vi "FTIR_multiple.vi"() -> ()   [LabVIEW 2021]
uses:
  <vilib>/express/express analysis/Spectral/Block/exnSpectralBlock spectral measurements PSD poly.vi
  <vilib>/express/express analysis/Spectral/Block/exnSpectralBlock spectral measurements PSD DDT.vi
  <vilib>/express/express analysis/Spectral/XNode/ExpressSpectralMeasurementsBlockNode.xnode
panel:
  out "Interferogram frequency":dbl[](array[numeric])
  out "Interferogram":dynamicdata(graph)
  out "FFT interferogram":dynamicdata(graph)
  out "Waveform signal":dynamicdata(graph)
  in  "Mirror 1 distance":dbl
  out "Phase":dbl[](array[numeric])
  out "size(s)":i32
  in  "Mirror speed":dbl(slide) scale=0.0..0.3
  out "Frequency 2":dbl[](array[numeric])
  out "Frequency 1":dbl[](array[numeric])
  out "Wavenumber":dbl[](array[numeric])
  in  "Wavelength":dbl[](array[numeric])
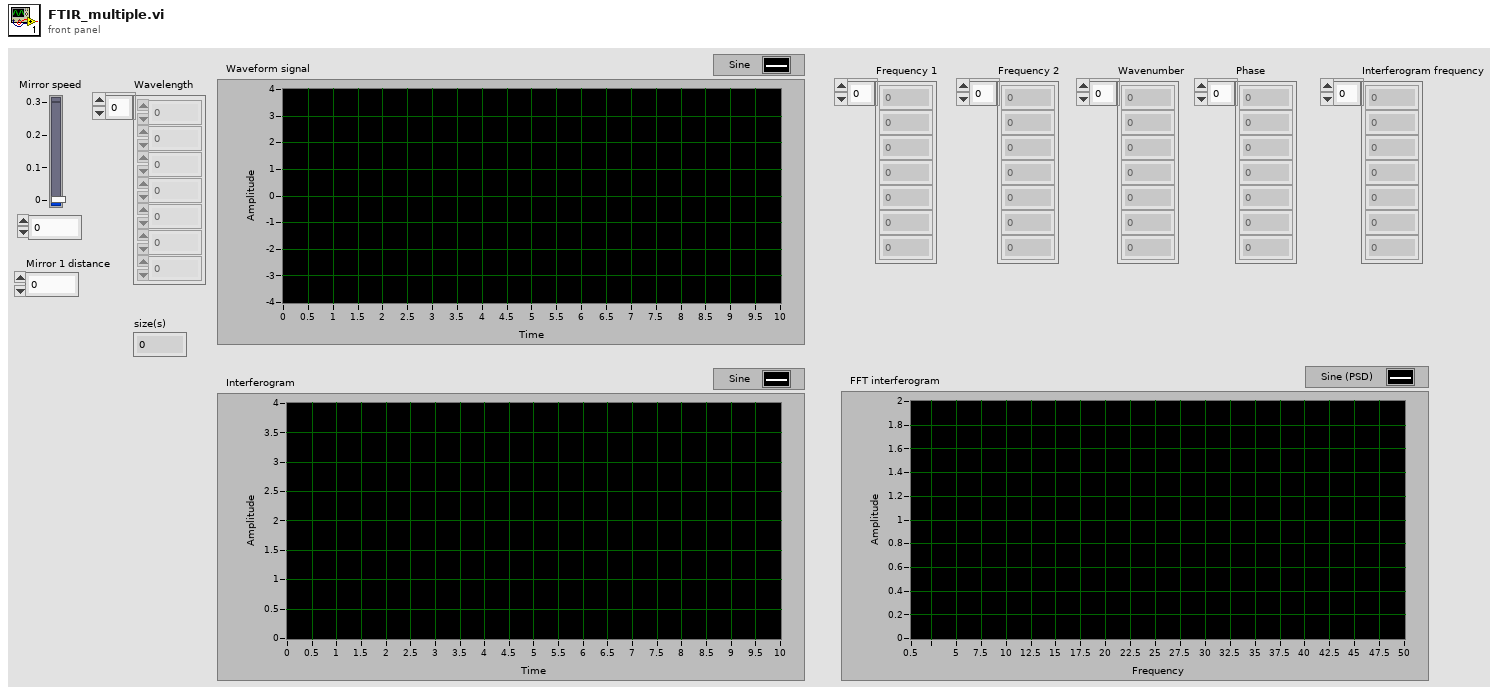
[diagram p1: front panel]
types:
  T1 = cluster{"averaging mode":u16, "weighting mode":u16, "number of averages":u32}
  T2 = cluster{"dB On (F)":bool, "unwrap phase (F)":bool, "convert to degree (F)":bool}
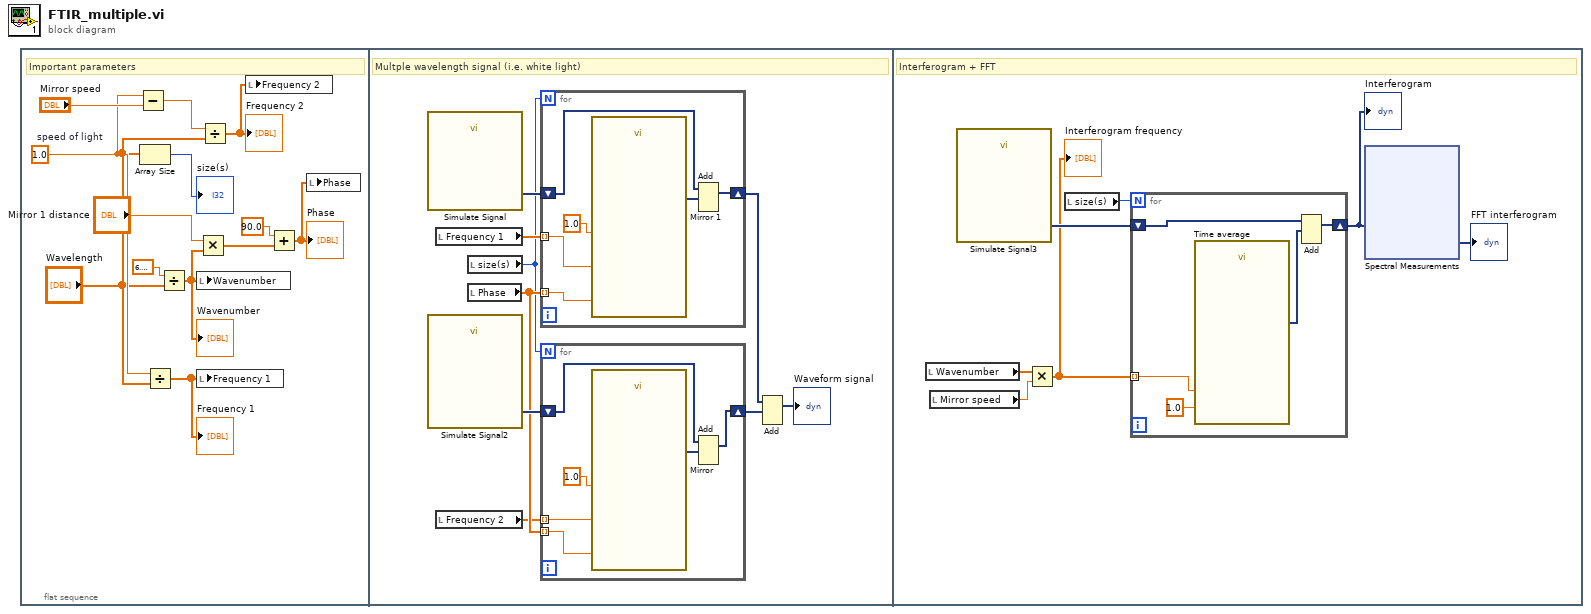
[diagram p0: block diagram]
diagram:
  n1 = flat-sequence {
    frame #0 {
      w11 = 1.0  # speed of light
      # "Important parameters"
      n2 = Subtract(x=w11, y="Mirror speed") -> (x-y=w13:dbl)
      n3 = Array Size(array="Wavelength") -> (size(s)=→"size(s)":i32)
      n4 = Divide(x=w11, y="Wavelength") -> (x/y=w6:dbl[])
      "Frequency 1" <- w6
      n5 = Divide(x=6.283185307179586, y="Wavelength") -> (x/y=w7:dbl[])
      "Wavenumber" <- w7
      n6 = local write "Wavenumber"(w7) -> ()
      n7 = local write "Frequency 1"(w6) -> ()
      n8 = Multiply(x="Mirror 1 distance", y=w7) -> (x*y=w9:dbl[])
      n9 = Divide(x=w13, y="Wavelength") -> (x/y=w5:dbl[])
      "Frequency 2" <- w5
      n10 = local write "Frequency 2"(w5) -> ()
      n11 = Add(x=90.0 ("y"), y=w9) -> (x+y=w2:dbl[])
      "Phase" <- w2
      n12 = local write "Phase"(w2) -> ()
    }
    frame #1 {
      # "Multple wavelength signal (i.e. white light)"
      n13 = call "Simulate Signal"() -> ("Sine"=w21:dynamicdata)  [unwired: 14 in, 1 out]
      n14 = call "Simulate Signal2"() -> ("Sine"=w20:dynamicdata)  [unwired: 14 in, 1 out]
      n15 = local read "Frequency 1"() -> (w22:dbl[])
      n16 = local read "Frequency 2"() -> (w17:dbl[])
      n17 = local read "size(s)"() -> (w18:i32)
      n18 = local read "Phase"() -> (w19:dbl[])
      n19 = for {
        N: w18 -> [_]
        tunnel: w22 -> [w34] mode=indexing
        tunnel: w19 -> [w33] mode=indexing
        shift-right: [w30] -> w16
        shift-left: w21 -> [w31]
        n20 = call "Mirror 1"("Frequency"=w34, "Amplitude"=1.0, "Phase"=w33) -> ("Sine"=w32:dynamicdata)  [unwired: 11 in, 1 out]
        n21 = Add(1:w32, 2:w31) -> (0:w30:dynamicdata)  [unwired: 1 in, 1 out]
      }
      n22 = for {
        N: w18 -> [_]
        shift-right: [w26] -> w15
        shift-left: w20 -> [w27]
        tunnel: w19 -> [w25] mode=indexing
        tunnel: w17 -> [w24] mode=indexing
        n23 = call "Mirror"("Frequency"=w24, "Amplitude"=1.0, "Phase"=w25) -> ("Sine"=w28:dynamicdata)  [unwired: 11 in, 1 out]
        n24 = Add(1:w28, 2:w27) -> (0:w26:dynamicdata)  [unwired: 1 in, 1 out]
      }
      n25 = Add(1:w15, 2:w16) -> (0:→"Waveform signal":dynamicdata)  [unwired: 1 in, 1 out]
    }
    frame #2 {
      # "Interferogram + FFT"
      n26 = local read "Wavenumber"() -> (w39:dbl[])
      n27 = local read "Mirror speed"() -> (w38:dbl)
      n28 = call "Simulate Signal3"() -> ("Sine"=w40:dynamicdata)  [unwired: 14 in, 1 out]
      n29 = Multiply(x=w39, y=w38) -> (x*y=w35:dbl[])
      "Interferogram frequency" <- w35
      n30 = local read "size(s)"() -> (w41:i32)
      n31 = for {
        N: w41 -> [_]
        shift-right: [w54] -> w36
        shift-left: w40 -> [w53]
        tunnel: w35 -> [w52] mode=indexing
        n32 = call "Time average"("Offset"=1.0, "Frequency"=w52) -> ("Sine"=w55:dynamicdata)  [unwired: 12 in, 1 out]
        n33 = Add(1:w55, 2:w53) -> (0:w54:dynamicdata)  [unwired: 1 in, 1 out]
      }
      "Interferogram" <- w36
      n34 = xnode "Spectral Measurements"("Signals"=w36) -> ("PSD"=→"FFT interferogram":dynamicdata)  [unwired: 1 in, 1 out]
    }
  }
